vi "mux6_1(3 wires)_separated.vi"(1 "Boolean array":bool[](array[boolean]), 4 "Mem_mapping in":u16[](array[numeric])) -> (8 "output array 11":bool[](array[boolean]))   [LabVIEW 2018, in "MB Relay.lvlib"]
uses:
  MB Relay.lvlib
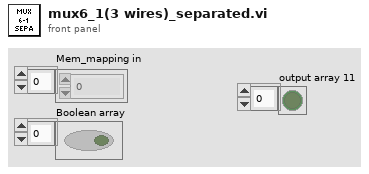
[diagram p1: front panel]
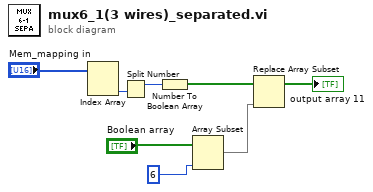
[diagram p0: block diagram]
diagram:
  n1 = Index Array(array="Mem_mapping in") -> (element #2=w7:u16)  [unwired: 2 in, 1 out]
  n2 = Split Number(x=w7) -> (hi(x)=w8:u8)  [unwired: 1 out]
  n3 = Number To Boolean Array(number=w8) -> (Boolean array=w3:bool[])
  n4 = Array Subset(array="Boolean array", length=6 ("index")) -> (w2:bool[])  [unwired: 1 in]
  n5 = Replace Array Subset(array=w3, new element=w2) -> (→"output array 11":bool[])  [unwired: 1 in]
